vi "LabJackU3_Global.vi"() -> ()   [LabVIEW 2019]
uses:
  temperature_status_LabJackU3.ctl
panel:
  out "LJU3_TEMP_ST":T1
  out "LJU3_ST":u32(colorbox)
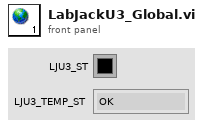
[diagram p1: front panel]
types:
  T1 = typedef "temperature_status_LabJackU3.ctl" = enum16{"OK", "UNKNOWN", "WARNING", "ERROR"}
diagram:
